vi "LVClass_CorrectionDataManager GetInteractionMatrixSize.vi"(0 "CorrectionDataManager in":refnum<class "CorrectionDataManager.lvclass">, 11 "error in (no error)":errorcluster) -> (4 "CorrectionDataManager out":refnum<class "CorrectionDataManager.lvclass">, 6 "# of valid actuators (nb col)":u32, 8 "2 time of valid sub pupil (nb line)":u32, 15 "error out":errorcluster)   [LabVIEW 2020, in "CorrectionDataManager.lvclass"]
doc: "Interaction matrix size getter.\n\n<B>corrdata_managerIn</B> : CorrDataManager object.\n<B>corrdata_managerOut</B> : CorrDataManager object.\n<B>size</B> : Size of interaction matrix."
uses:
  CorrectionDataManager.lvclass
  Controls/Point2D.ctl
  CorrectionDataManager.lvclass/CorrectionDataManager.ctl
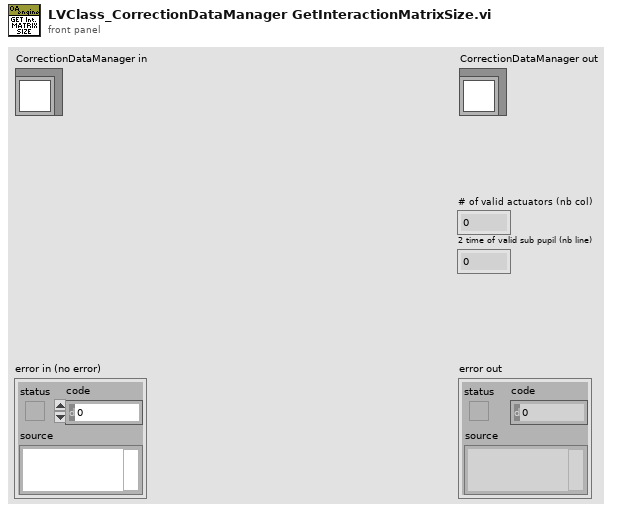
[diagram p1: front panel]
types:
  T1 = typedef "Point2D.ctl" = cluster{"X":u32, "Y":u32}
  T2 = typedef "ClassID.ctl" = i64
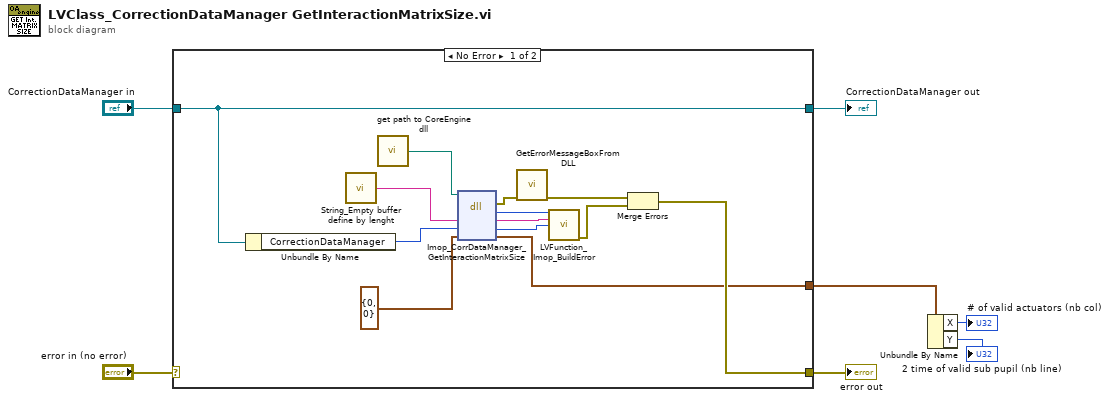
[diagram p0: block diagram]
diagram:
  n1 = case shown="No Error" "error in (no error)" {
    selector: "error in (no error)" -> [_ w22]
    tunnel: [w12 w22] -> w6
    tunnel: [w13 w21] -> w7
    tunnel: "CorrectionDataManager in" -> [w13 w21]
    tunnel: [w9 _] -> w1
    frame No Error {
      n2 = Unbundle By Name(w13) -> ("CorrectionDataManager"=w11:T2)
      n3 = call "String_Empty buffer define by lenght.vi"() -> ("Empty buffer"=w18:string)  [unwired: 1 in]
      n4 = call "get path to CoreEngine dll.vi"() -> ("path to wavekit library"=w17:path)  [unwired: 14 in, 1 out]
      n5 = dll-call lib="D:/soft/HASO_v3/SVN_trunk/ImOpCoreEngine4_LV2011/DLLs/c_interface_vc100.dll" fn="Imop_CorrDataManager_GetInteractionMatrixSize"(path in=w17, "message"=w18, "WavefrontCorrection"=w11, "size"=T1 {"X"=0, "Y"=0}) -> (error out=w16:errorcluster, "return type"=w20:i32, "message"=w19:string, "WavefrontCorrection"=w8:i64, "size"=w9:T1)  [unwired: 2 in, 1 out]
      n6 = call "GetErrorMessageBoxFromDLL.vi"("error IN"=w16) -> ("error OUT"=w15:errorcluster)  [unwired: 10 in]
      n7 = call "LVFunction_Imop_BuildError.vi"("code"=w20, "String to Prepend to source (\"\")"=w19, "Adresse"=w8) -> ("error out"=w14:errorcluster)  [unwired: 12 in]
      n8 = Merge Errors(w15, w14) -> (w12:errorcluster)
    }
    frame Error {
    }
  }
  "error out" <- w6
  "CorrectionDataManager out" <- w7
  n9 = Unbundle By Name(w1) -> ("X"=→"# of valid actuators (nb col)":u32, "Y"=→"2 time of valid sub pupil (nb line)":u32)
